vi "一体站氨氮总磷流程质控自动启动.vi"(6 "CODMn量程切换":enum32{"H", "L", "AUTO"}(ring)=enum."AUTO", 8 "总磷量程切换":enum32{"H", "L", "AUTO"}(ring)=enum."AUTO", 9 "总氮量程切换":enum32{"H", "L", "AUTO"}(ring)=enum."AUTO", 10 "氨氮量程切换":enum32{"H", "L", "AUTO"}(ring)=enum."AUTO", 11 "参数":T1={"是否启用仪器"=FALSE, "CODMn"={"启动测量模式"={"测量模式"=enum."水样测量"}, "确定按钮"=TRUE}, "启动模块"={"氨氮"=FALSE, "总磷"=FALSE, "总氮"=FALSE, "CODMn"=FALSE, "CODCr"=FALSE}, "常规启动"=FALSE, "直接启动"=FALSE}) -> ()   [LabVIEW 2016]
panel:
  out "枚举":enum16{"初始化", "采配水启动", "等待", "配水", "排水", "结束"}(ring)
  out "枚举 2":enum16{"初始化", "采配水启动", "等待", "配水", "排水", "结束"}(ring)
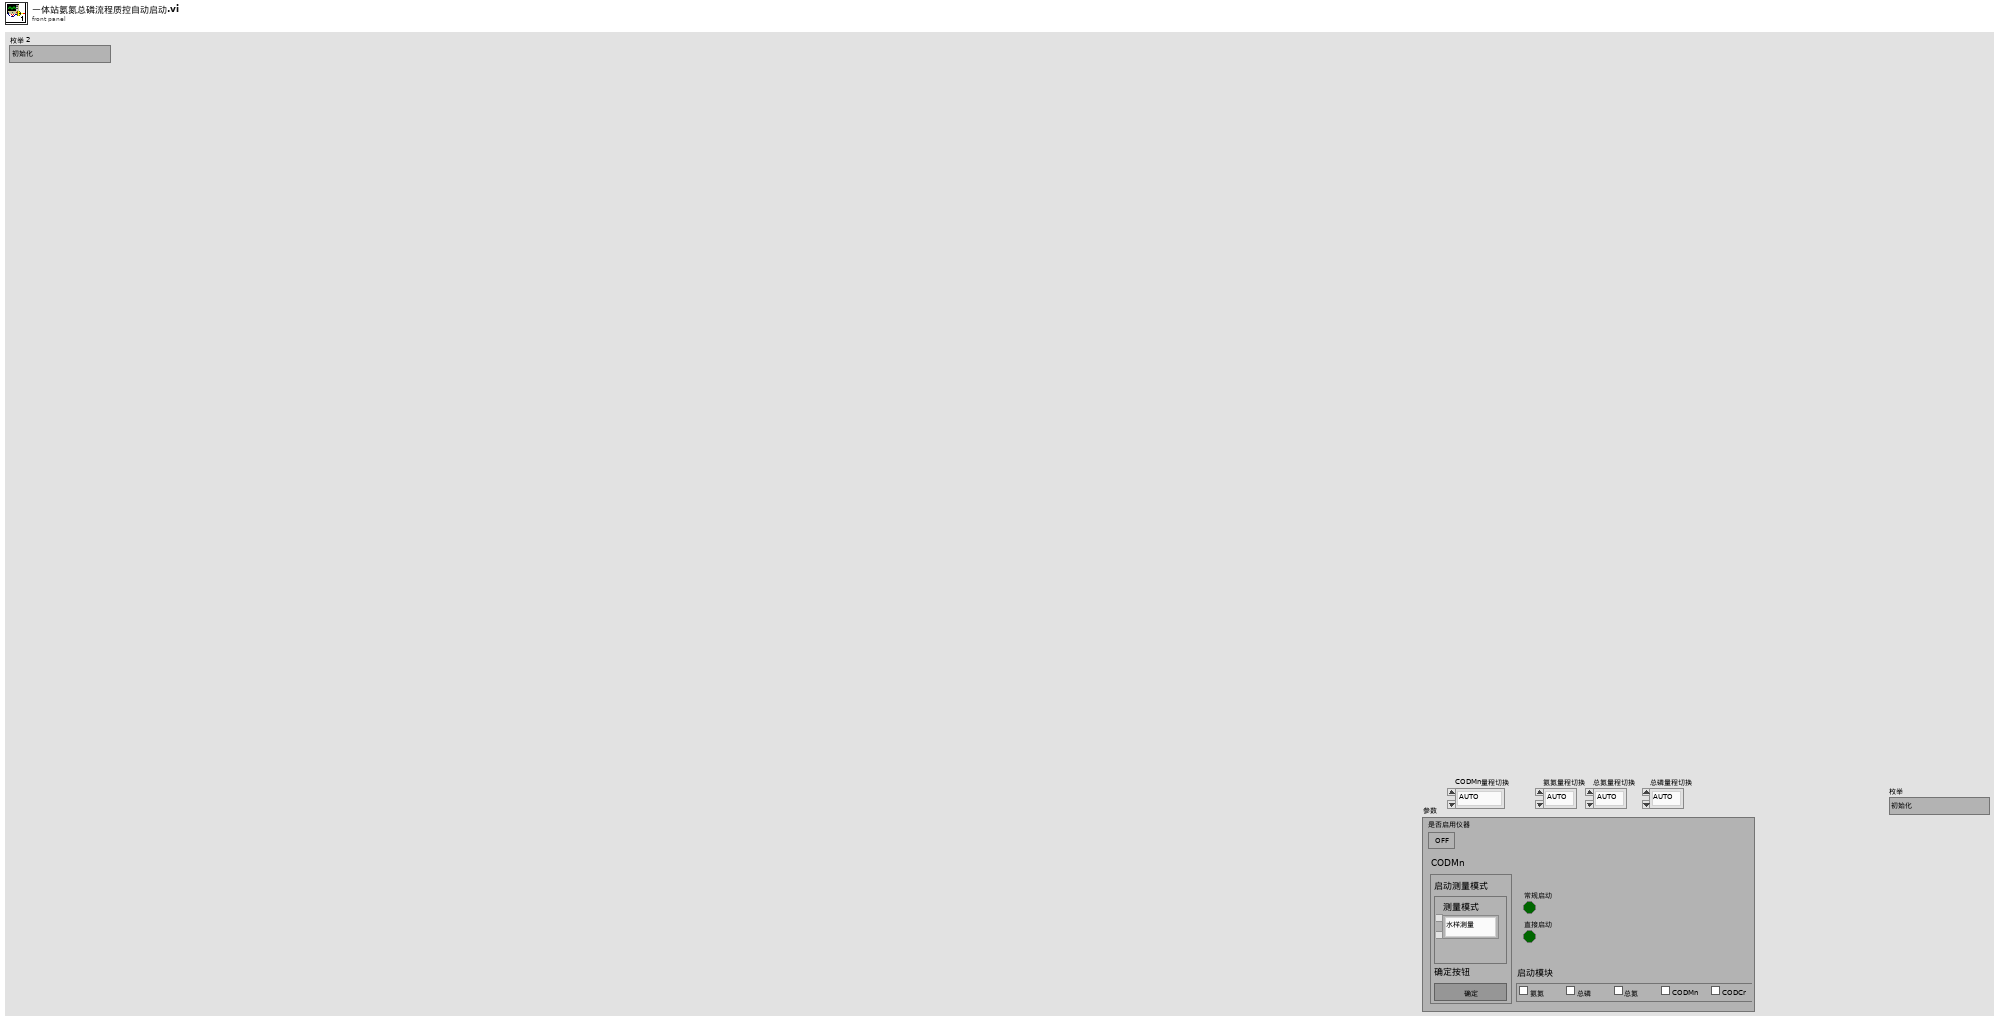
[diagram p1: front panel]
types:
  T1 = cluster{"是否启用仪器":bool, "CODMn":cluster{"启动测量模式":cluster{"测量模式":enum16{"水样测量", "标样核查", "加标回收", "平行样", "校零", "校标"}}, "确定按钮":bool}, "启动模块":cluster{"氨氮":bool, "总磷":bool, "总氮":bool, "CODMn":bool, "CODCr":bool}, "常规启动":bool, "直接启动":bool}
  T2 = cluster{"命令":string, cluster{"starting address":u16, "holding register value":u16}}
  T3 = cluster{"R0":i16, "R1":i16, "R2":i16, "R3":i16, "R4":i16, "R5":i16, "R6":i16, "R7":i16, "R8":i16, "R9":i16, "R10":i16, "R11":i16, "R12":i16, "R13":i16, "R14":i16, "R15":i16, "R16":i16, "R17":i16, "R18":i16, "R19":i16, "R20":i16, "R21":i16, "R22":i16, "R23":i16, "R24":i16, "R25":i16, "R26":i16, "R27":i16, "R28":i16, "R29":i16, "R30":i16, "R31":i16, "R32":i16, "R33":i16, "R34":i16, "R35":i16, "R36":i16, "R37":i16, "R38":i16, "R39":i16, "R40":i16, "R41":i16, "R42":i16, "R43":i16, "R44":i16, "R45":i16, "R46":i16, "R47":i16, "R48":i16, "R49":i16, "R50":i16, "R51":i16, "R52":i16, "R53":i16, "R54":i16, "R55":i16, "R56":i16}
  T4 = enum32{"Bad", "Idle", "Run top level", "Running"}
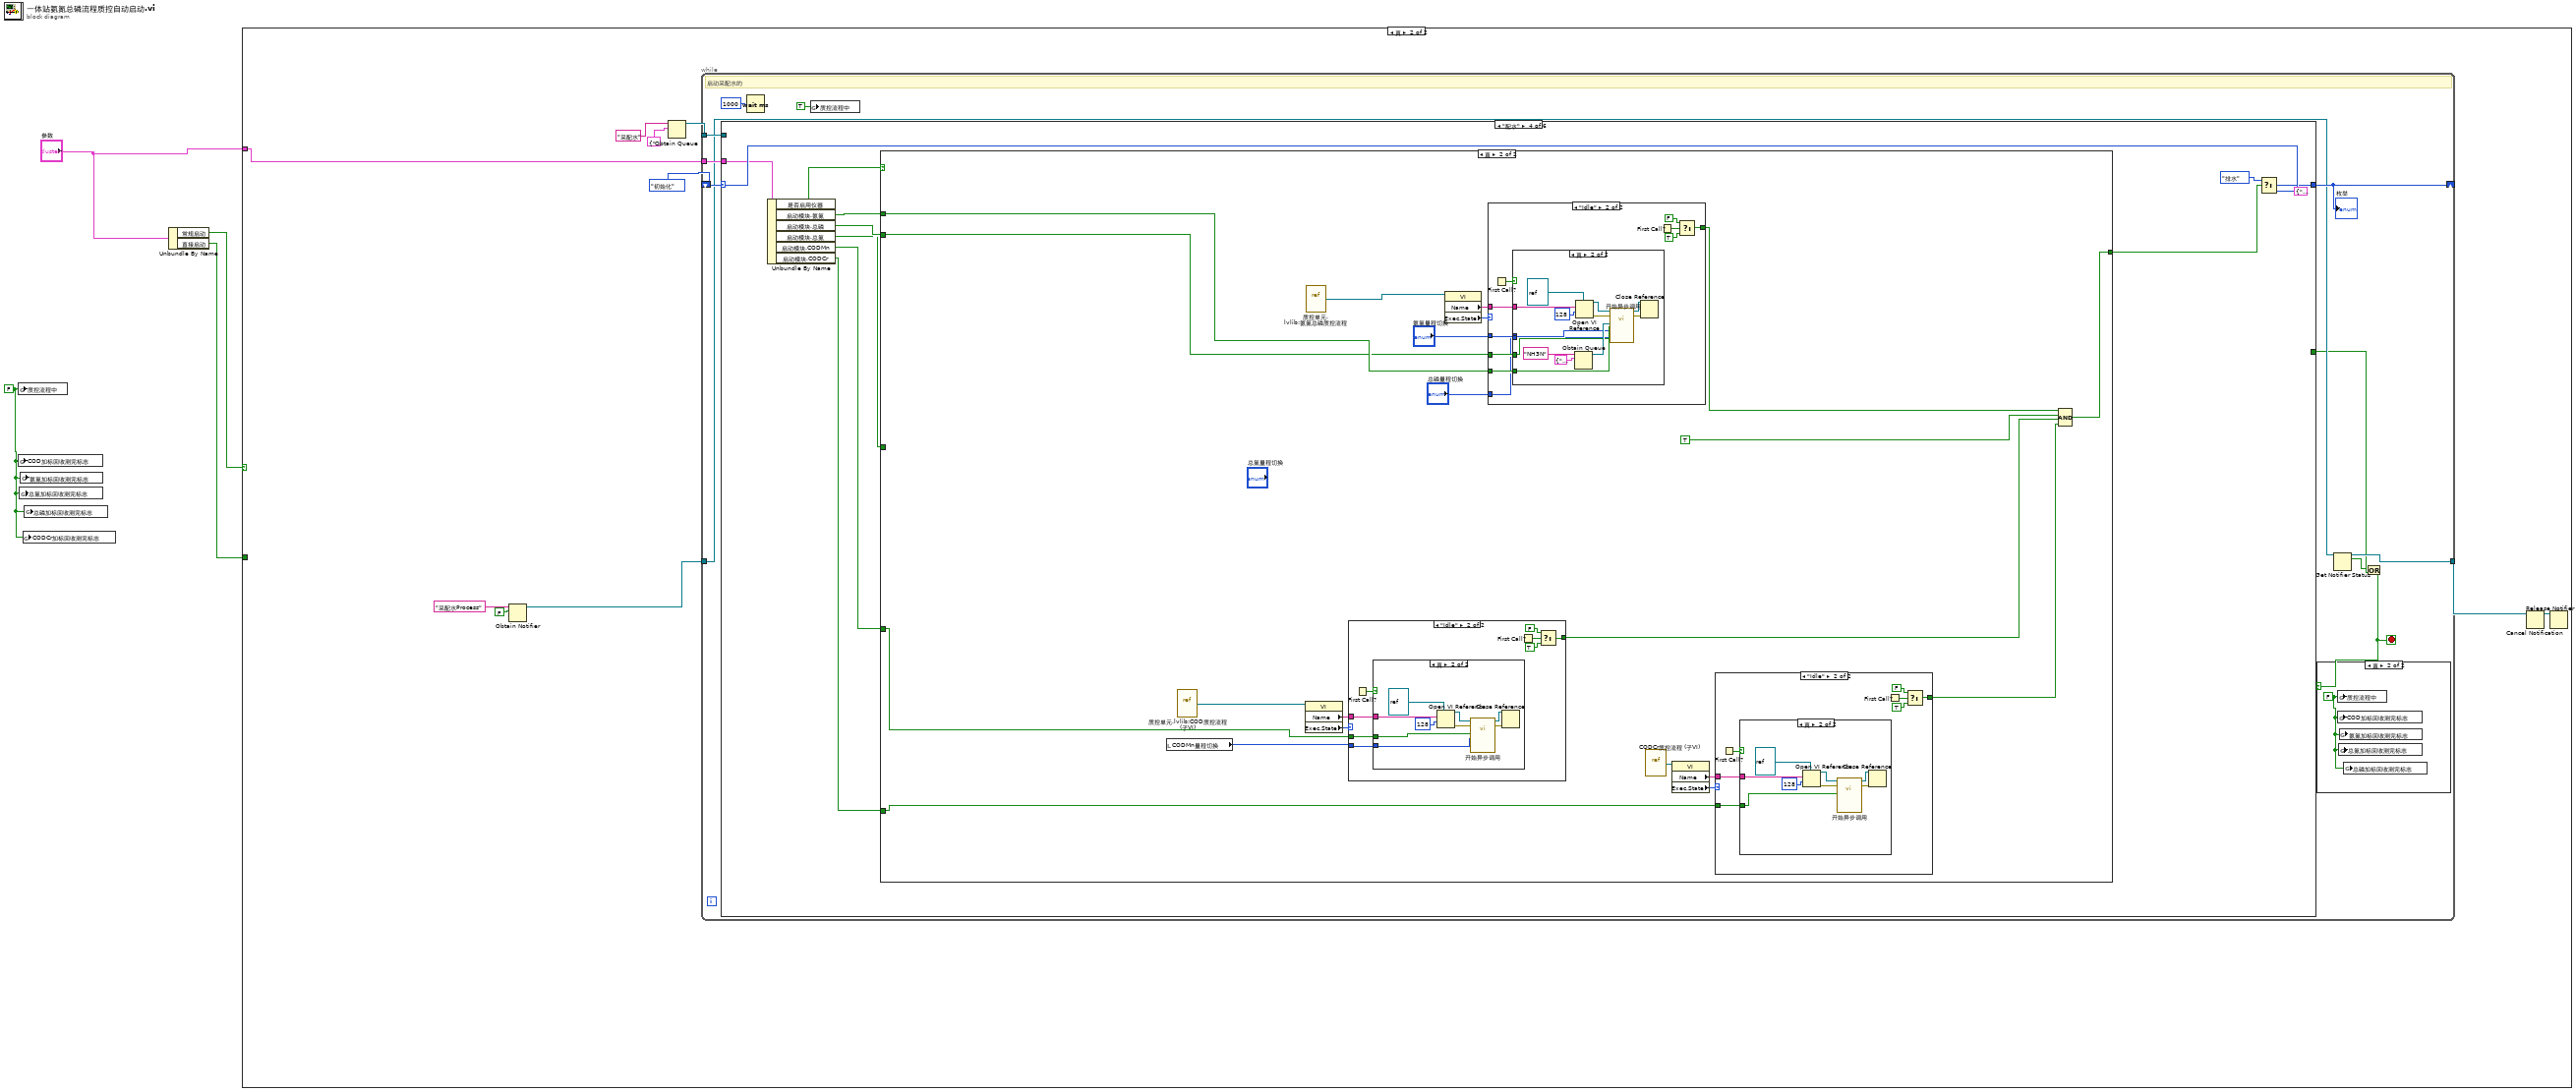
[diagram p0: block diagram]
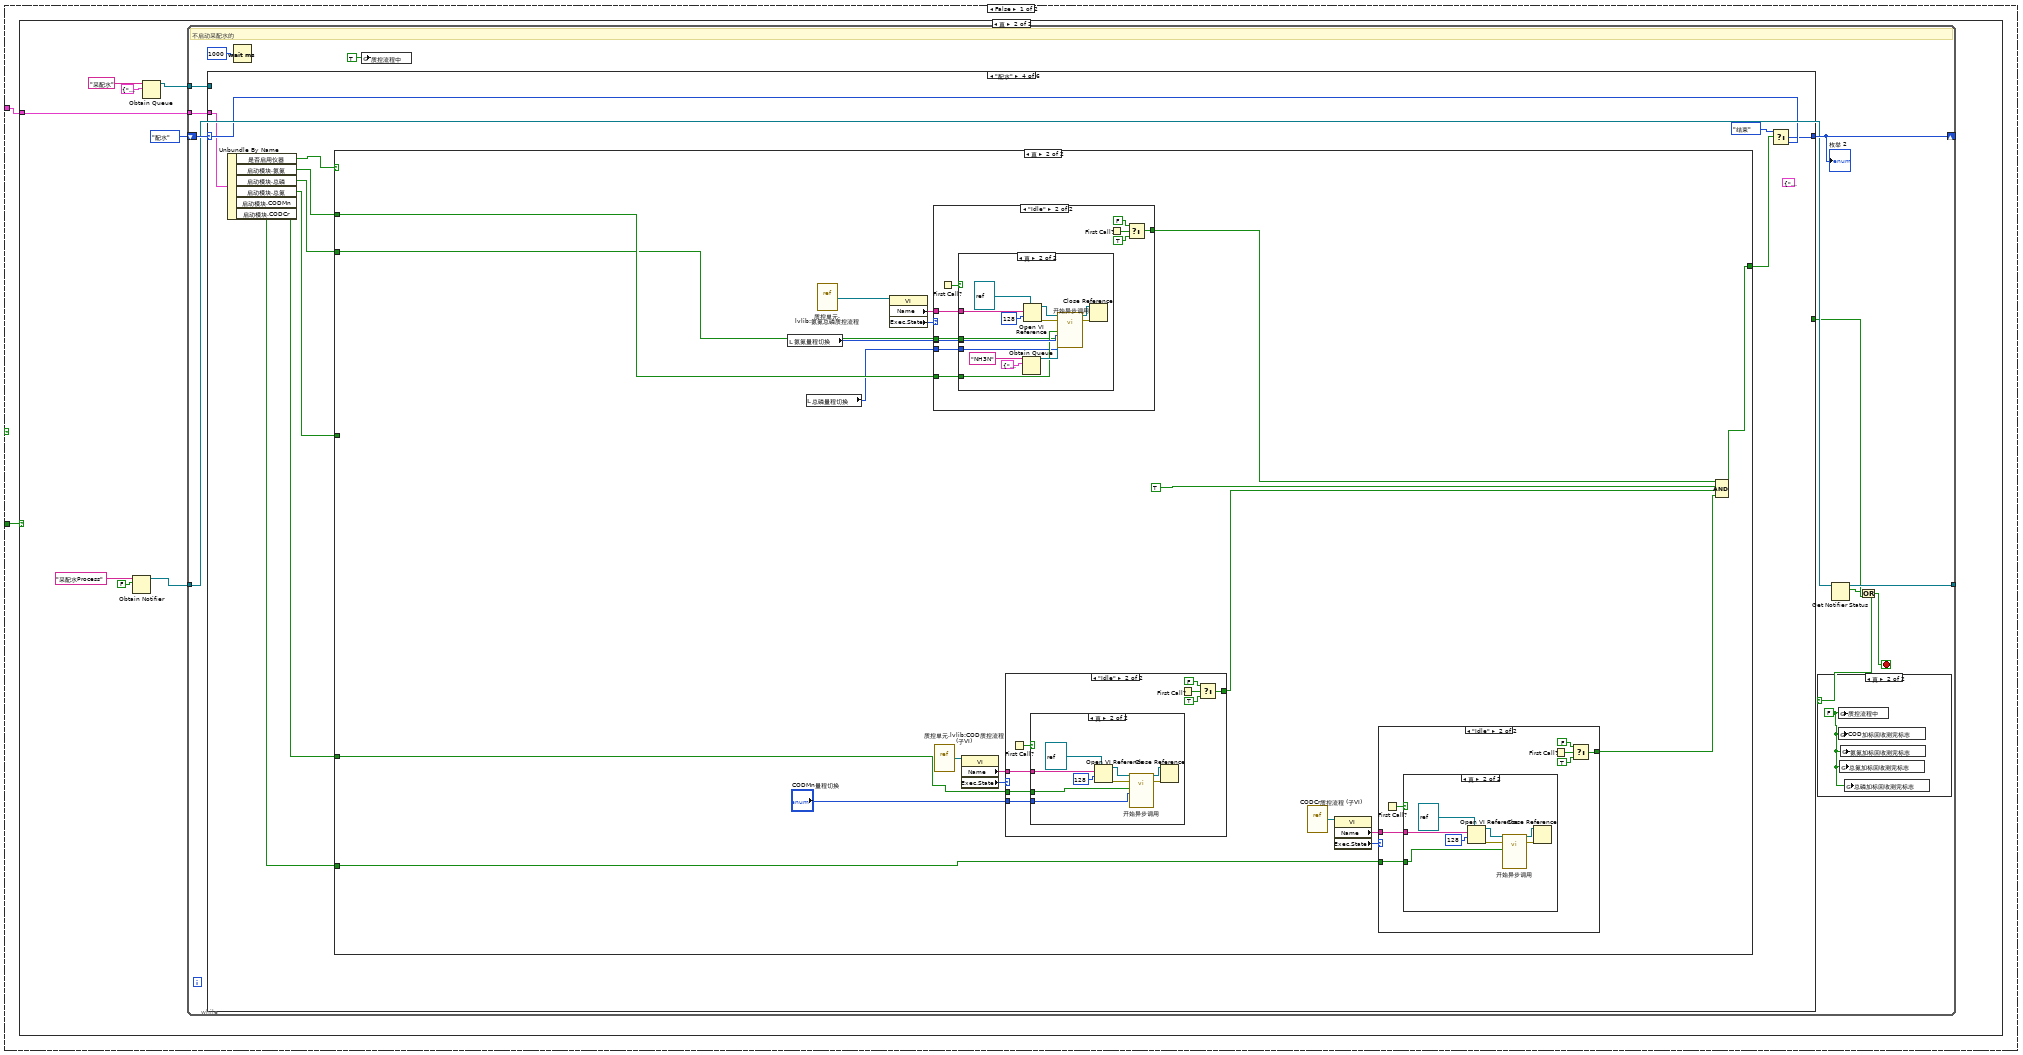
[diagram p2: hidden frame]
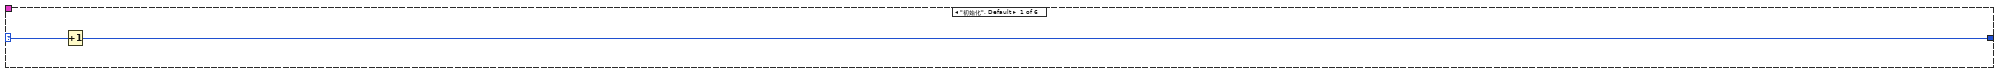
[diagram p5: hidden frame]
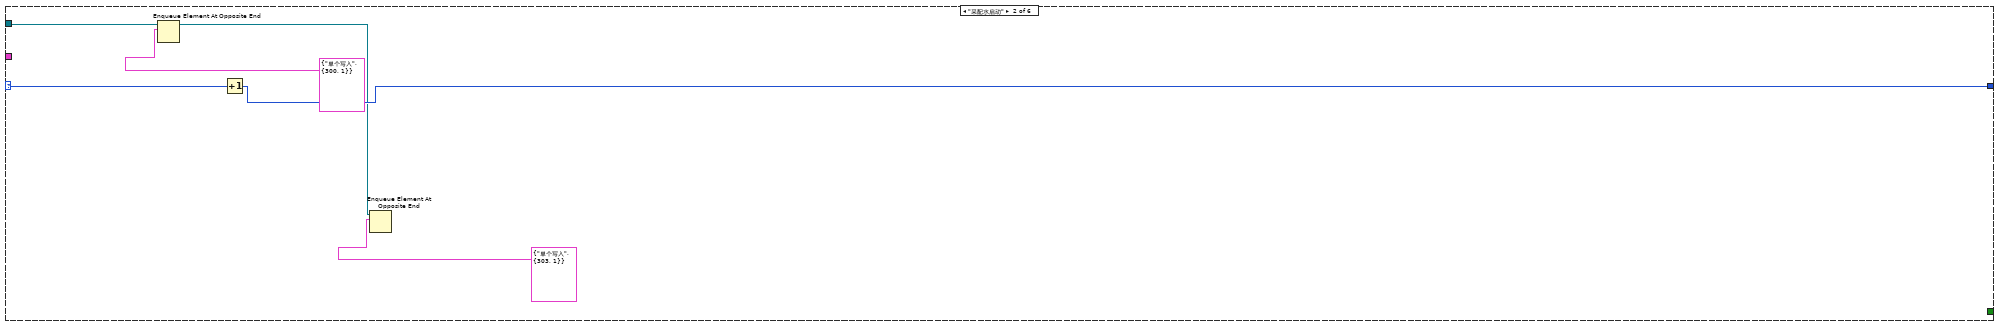
[diagram p6: hidden frame]
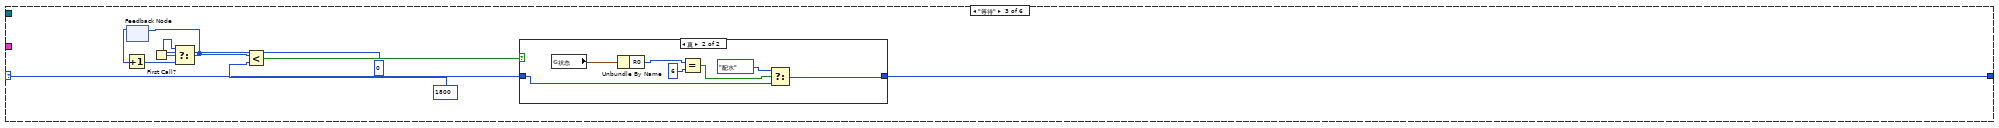
[diagram p7: hidden frame]
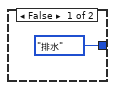
[diagram p8: hidden frame]
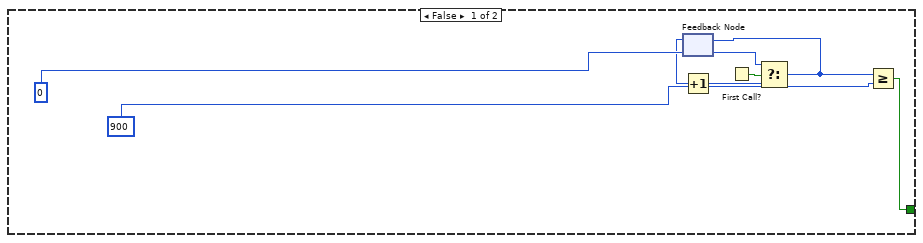
[diagram p9: hidden frame]
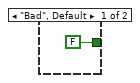
[diagram p10: hidden frame]
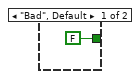
[diagram p12: hidden frame]
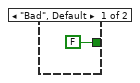
[diagram p14: hidden frame]
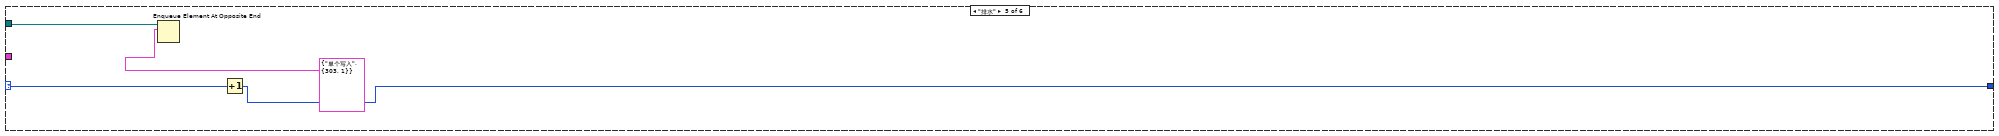
[diagram p16: hidden frame]
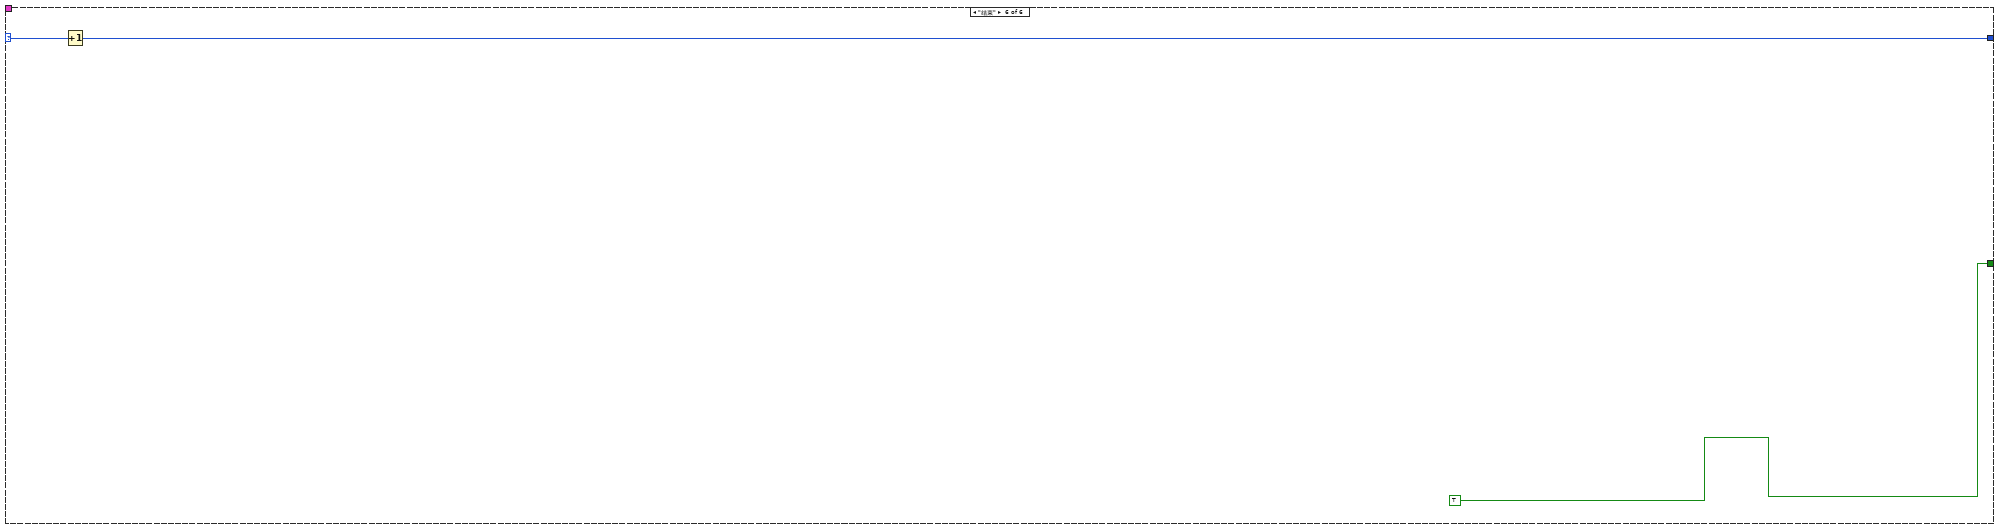
[diagram p17: hidden frame]
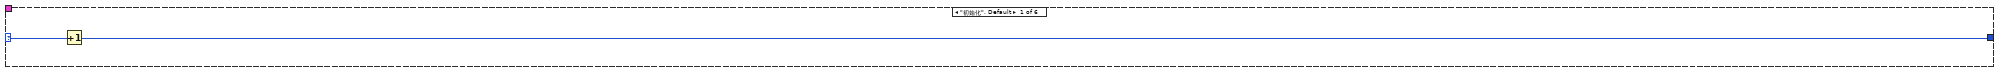
[diagram p19: hidden frame]
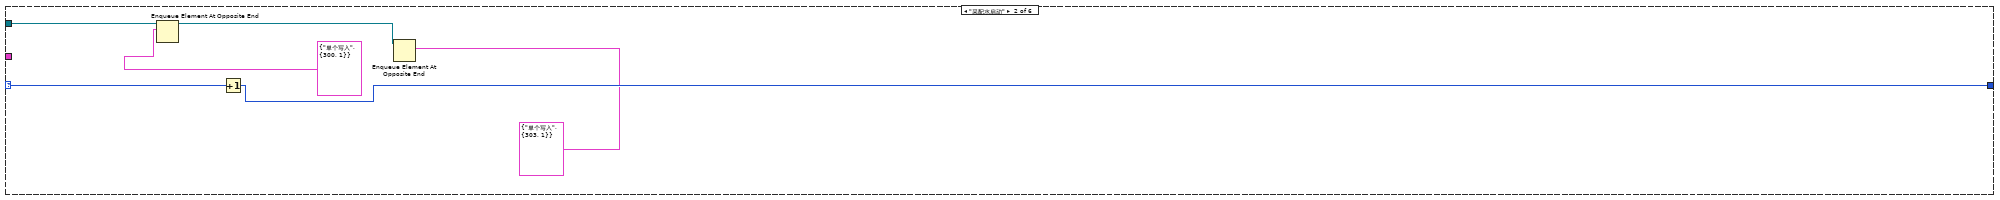
[diagram p20: hidden frame]
diagram:
  w1 = FALSE ("质控流程中")
  n1 = global write "质控测完标志全局 1.vi" "质控流程中"(w1) -> ()
  n2 = global write "质控测完标志全局 1.vi" "COD加标回收测完标志"(w1) -> ()
  n3 = global write "质控测完标志全局 1.vi" "总氮加标回收测完标志"(w1) -> ()
  n4 = global write "质控测完标志全局 1.vi" "氨氮加标回收测完标志"(w1) -> ()
  n5 = global write "质控测完标志全局 1.vi" "CODCr加标回收测完标志"(w1) -> ()
  n6 = global write "质控测完标志全局 1.vi" "总磷加标回收测完标志"(w1) -> ()
  n7 = Unbundle By Name("参数") -> ("常规启动"=w3:bool, "直接启动"=w2:bool)
  n8 = case shown="真" w3 {
    tunnel: "参数" -> [w5 w157]
    tunnel: w2 -> [w6 _]
    frame False {
      n9 = case shown="真" w6 {
        tunnel: w5 -> [_ w13]
        frame False {
        }
        frame True {
          n10 = Obtain Notifier(name (unnamed)="采配水Process" ("名称（未命名）"), notification data type=FALSE) -> (notifier out=w7:refnum<notifier>)  [unwired: 2 in, 2 out]
          n11 = Obtain Queue(name (unnamed)="采配水" ("名称（未命名）"), element data type=cluster{"命令":string, "数据":variant} {"命令"="", "数据"=variant}) -> (queue out=w10:refnum<queue>)  [unwired: 3 in, 2 out]
          n12 = while {
            tunnel: w10 -> [w25]
            shift-right: [w23] -> _
            shift-left: enum16{"初始化", "采配水启动", "等待", "配水", "排水", "结束"}."配水" ("枚举") -> [w24]
            tunnel: w13 -> [w21]
            tunnel: w7 -> [w20]
            tunnel: [w19] -> _
            stop <- w16 stop-if-true
            # "不启动采配水的"
            n13 = case shown="\"配水\"" w24 {
              selector: w24 -> [w28 w32 w41 w61 w151 w156]
              tunnel: w25 -> [_ w33 _ _ w152 _]
              tunnel: [w27 w31 w40 w60 w150 w155] -> w23
              tunnel: [_ _ _ _ _ TRUE] -> w18
              tunnel: w21 -> [_ _ _ w57 _ _]
              frame "初始化", Default {
                n14 = Increment(x=w28) -> (x+1=w27:enum16{"初始化", "采配水启动", "等待", "配水", "排水", "结束"})
              }
              frame "采配水启动" {
                n15 = Enqueue Element At Opposite End(queue=w33, element=T2 {"命令"="单个写入", {"starting address"=300, "holding register value"=1}} ("元素")) -> (queue out=w29:refnum<queue>)  [unwired: 2 in, 2 out]
                n16 = Increment(x=w32) -> (x+1=w31:enum16{"初始化", "采配水启动", "等待", "配水", "排水", "结束"})
                n17 = Enqueue Element At Opposite End(queue=w29, element=T2 {"命令"="单个写入", {"starting address"=303, "holding register value"=1}} ("元素")) -> ()  [unwired: 2 in, 3 out]
              }
              frame "等待" {
                n18 = feedback #1() -> (w37:i32)  [unwired: 1 in]
                n19 = Increment(x=w37) -> (x+1=w36:i32)
                n20 = First Call?() -> (First Call?: T/F=w38:bool)
                n21 = Select(t=0, s=w38, f=w36) -> (s? t:f=w35:i32)
                n22 = feedback-in #1(w35) -> ()
                n23 = Less?(x=w35, y=1800) -> (x < y?=w42:bool)
                n24 = case shown="真" w42 {
                  tunnel: w41 -> [_ w47]
                  tunnel: [enum16{"初始化", "采配水启动", "等待", "配水", "排水", "结束"}."排水" ("枚举") w46] -> w40
                  frame False {
                  }
                  frame True {
                    n25 = global read "与采配水交互全局.vi" "状态"() -> (w45:T3)
                    n26 = Unbundle By Name(w45) -> ("R0"=w51:i16)
                    n27 = Equal?(x=w51, y=i16 6) -> (x = y?=w49:bool)
                    n28 = Select(t=enum16{"初始化", "采配水启动", "等待", "配水", "排水", "结束"}."配水" ("枚举"), s=w49, f=w47) -> (s? t:f=w46:enum16{"初始化", "采配水启动", "等待", "配水", "排水", "结束"})
                  }
                }
              }
              frame "配水" {
                (unwired) cluster{"命令":string, "data":variant} {"命令"="启动", "data"=variant(cluster{"站号":u16, "控制命令输出":u16[]} {"站号"=1, "控制命令输出"=[256, 0]})} ("元素")
                n29 = Unbundle By Name(w57) -> ("是否启用仪器"=w59:bool, "启动模块.氨氮"=w55:bool, "启动模块.总磷"=w56:bool, "启动模块.总氮"=w53:bool, "启动模块.CODMn"=w54:bool, "启动模块.CODCr"=w52:bool)
                n30 = case shown="真" w59 {
                  tunnel: [w63 w90] -> w58
                  tunnel: w56 -> [_ w71]
                  tunnel: w55 -> [_ w86]
                  tunnel: w54 -> [_ w76]
                  tunnel: w53 -> [_ _]
                  tunnel: w52 -> [_ w73]
                  frame False {
                    n31 = feedback #2() -> (w67:i32)  [unwired: 1 in]
                    n32 = Increment(x=w67) -> (x+1=w66:i32)
                    n33 = First Call?() -> (First Call?: T/F=w68:bool)
                    n34 = Select(t=0, s=w68, f=w66) -> (s? t:f=w64:i32)
                    n35 = feedback-in #2(w64) -> ()
                    n36 = Greater Or Equal?(x=w64, y=900) -> (x >= y?=w63:bool)
                  }
                  frame True {
                    n37 = local read "氨氮量程切换"() -> (w84:enum32{"H", "L", "AUTO"})
                    n38 = local read "总磷量程切换"() -> (w70:enum32{"H", "L", "AUTO"})
                    n39 = vi-ref "质控单元.lvlib:氨氮总磷质控流程.vi"() -> (w88:refnum<vi>)
                    n40 = property class="VI"(reference=w88) -> ("Name"=w89:string, "Exec.State"=w87:T4)  [unwired: 1 in, 2 out]
                    n41 = case shown="\"Idle\"" w87 {
                      tunnel: w89 -> [_ w135]
                      tunnel: w86 -> [_ w134]
                      tunnel: [FALSE w129] -> w85
                      tunnel: w84 -> [_ w128]
                      tunnel: w71 -> [_ w127]
                      tunnel: w70 -> [_ w126]
                      frame "Bad", Default {
                      }
                      frame "Idle" {
                        n42 = First Call?() -> (First Call?: T/F=w133:bool)
                        n43 = case shown="真" w133 {
                          tunnel: w135 -> [_ w148]
                          tunnel: w134 -> [_ w138]
                          tunnel: w128 -> [_ w139]
                          tunnel: w127 -> [_ w137]
                          tunnel: w126 -> [_ w136]
                          frame False {
                          }
                          frame True {
                            n44 = Obtain Queue(name (unnamed)="NH3N" ("名称（未命名）"), element data type=cluster{"命令":string, "data":variant} {"命令"="", "data"=variant}) -> (queue out=w140:refnum<queue>)  [unwired: 3 in, 2 out]
                            n45 = Open VI Reference(type specifier VI Refnum (for type only)=refnum<vi> refnum ("类型说明符VI引用句柄（仅用于类型）"), vi path=w148, options=128 ("选项")) -> (vi reference=w149:refnum<vi>, error out=w145:errorcluster)  [unwired: 3 in]
                            n46 = call-by-ref "开始异步调用"(reference=w149, error in=w145, "队列输入"=w140, "氨氮"=w138, "氨氮量程切换"=w139, "总磷"=w137, "总磷量程切换"=w136) -> (reference out=w147:refnum<vi>, error out=w146:errorcluster)  [unwired: 8 in, 3 out]
                            n47 = Close Reference(reference=w147, error in (no error)=w146) -> ()  [unwired: 1 out]
                          }
                        }
                        n48 = First Call?() -> (First Call?: T/F=w132:bool)
                        n49 = Select(t=FALSE, s=w132, f=TRUE) -> (s? t:f=w129:bool)
                      }
                    }
                    n50 = vi-ref "质控单元.lvlib:COD质控流程 (子VI).vi"() -> (w81:refnum<vi>)
                    n51 = property class="VI"(reference=w81) -> ("Name"=w82:string, "Exec.State"=w80:T4)  [unwired: 1 in, 2 out]
                    n52 = case shown="\"Idle\"" w80 {
                      tunnel: w82 -> [_ w115]
                      tunnel: [FALSE w110] -> w74
                      tunnel: "CODMn量程切换" -> [_ w109]
                      tunnel: w76 -> [_ w108]
                      frame "Bad", Default {
                      }
                      frame "Idle" {
                        n53 = First Call?() -> (First Call?: T/F=w114:bool)
                        n54 = case shown="真" w114 {
                          tunnel: w115 -> [_ w123]
                          tunnel: w109 -> [_ w116]
                          tunnel: w108 -> [_ w117]
                          frame False {
                          }
                          frame True {
                            n55 = Open VI Reference(type specifier VI Refnum (for type only)=refnum<vi> refnum ("类型说明符VI引用句柄（仅用于类型）"), vi path=w123, options=128 ("选项")) -> (vi reference=w124:refnum<vi>, error out=w120:errorcluster)  [unwired: 3 in]
                            n56 = call-by-ref "开始异步调用"(reference=w124, error in=w120, "CODMn量程切换"=w116, "COD"=w117) -> (reference out=w122:refnum<vi>, error out=w121:errorcluster)  [unwired: 8 in, 2 out]
                            n57 = Close Reference(reference=w122, error in (no error)=w121) -> ()  [unwired: 1 out]
                          }
                        }
                        n58 = First Call?() -> (First Call?: T/F=w113:bool)
                        n59 = Select(t=FALSE, s=w113, f=TRUE) -> (s? t:f=w110:bool)
                      }
                    }
                    n60 = vi-ref "CODCr质控流程 (子VI).vi"() -> (w78:refnum<vi>)
                    n61 = property class="VI"(reference=w78) -> ("Name"=w79:string, "Exec.State"=w77:T4)  [unwired: 1 in, 2 out]
                    n62 = case shown="\"Idle\"" w77 {
                      tunnel: w79 -> [_ w98]
                      tunnel: [FALSE w93] -> w72
                      tunnel: w73 -> [_ w92]
                      frame "Bad", Default {
                      }
                      frame "Idle" {
                        n63 = First Call?() -> (First Call?: T/F=w97:bool)
                        n64 = case shown="真" w97 {
                          tunnel: w98 -> [_ w105]
                          tunnel: w92 -> [_ w99]
                          frame False {
                          }
                          frame True {
                            n65 = Open VI Reference(type specifier VI Refnum (for type only)=refnum<vi> refnum ("类型说明符VI引用句柄（仅用于类型）"), vi path=w105, options=128 ("选项")) -> (vi reference=w106:refnum<vi>, error out=w102:errorcluster)  [unwired: 3 in]
                            n66 = call-by-ref "开始异步调用"(reference=w106, error in=w102, "CODCr"=w99) -> (reference out=w104:refnum<vi>, error out=w103:errorcluster)  [unwired: 9 in, 2 out]
                            n67 = Close Reference(reference=w104, error in (no error)=w103) -> ()  [unwired: 1 out]
                          }
                        }
                        n68 = First Call?() -> (First Call?: T/F=w96:bool)
                        n69 = Select(t=FALSE, s=w96, f=TRUE) -> (s? t:f=w93:bool)
                      }
                    }
                    n70 = Compound Arithmetic op=AND ("复合运算")(w85, TRUE, w74, w72) -> (w90:bool)
                  }
                }
                n71 = Select(t=enum16{"初始化", "采配水启动", "等待", "配水", "排水", "结束"}."结束" ("枚举"), s=w58, f=w61) -> (s? t:f=w60:enum16{"初始化", "采配水启动", "等待", "配水", "排水", "结束"})
              }
              frame "排水" {
                n72 = Enqueue Element At Opposite End(queue=w152, element=T2 {"命令"="单个写入", {"starting address"=303, "holding register value"=1}} ("元素")) -> ()  [unwired: 2 in, 3 out]
                n73 = Increment(x=w151) -> (x+1=w150:enum16{"初始化", "采配水启动", "等待", "配水", "排水", "结束"})
              }
              frame "结束" {
                n74 = Increment(x=w156) -> (x+1=w155:enum16{"初始化", "采配水启动", "等待", "配水", "排水", "结束"})
              }
            }
            "枚举 2" <- w23
            n75 = Wait (ms)(milliseconds to wait=u32 1000 ("等待时间（毫秒）")) -> ()  [unwired: 1 out]
            n76 = global write "质控测完标志全局 1.vi" "质控流程中"(TRUE ("质控流程中")) -> ()
            n77 = Get Notifier Status(notifier=w20) -> (notifier out=w19:refnum<notifier>, current notification=w17:bool)  [unwired: 1 in, 3 out]
            n78 = Or(x=w17, y=w18) -> (x .or. y?=w16:bool)
            n79 = case shown="真" w16 {
              frame False {
              }
              frame True {
                w26 = FALSE ("质控流程中")
                n80 = global write "质控测完标志全局 1.vi" "质控流程中"(w26) -> ()
                n81 = global write "质控测完标志全局 1.vi" "COD加标回收测完标志"(w26) -> ()
                n82 = global write "质控测完标志全局 1.vi" "总氮加标回收测完标志"(w26) -> ()
                n83 = global write "质控测完标志全局 1.vi" "氨氮加标回收测完标志"(w26) -> ()
                n84 = global write "质控测完标志全局 1.vi" "总磷加标回收测完标志"(w26) -> ()
              }
            }
          }
        }
      }
    }
    frame True {
      n85 = Obtain Notifier(name (unnamed)="采配水Process" ("名称（未命名）"), notification data type=FALSE) -> (notifier out=w160:refnum<notifier>)  [unwired: 2 in, 2 out]
      n86 = Obtain Queue(name (unnamed)="采配水" ("名称（未命名）"), element data type=cluster{"命令":string, "数据":variant} {"命令"="", "数据"=variant}) -> (queue out=w164:refnum<queue>)  [unwired: 3 in, 2 out]
      n87 = while {
        tunnel: w164 -> [w177]
        shift-right: [w175] -> _
        shift-left: enum16{"初始化", "采配水启动", "等待", "配水", "排水", "结束"}."初始化" ("枚举") -> [w176]
        tunnel: w157 -> [w173]
        tunnel: w160 -> [w172]
        tunnel: [w171] -> w159
        stop <- w168 stop-if-true
        # "启动采配水的"
        n88 = case shown="\"配水\"" w176 {
          selector: w176 -> [w180 w184 w193 w213 w303 w308]
          tunnel: w177 -> [_ w185 _ _ w304 _]
          tunnel: [w179 w183 w192 w212 w302 w307] -> w175
          tunnel: [_ _ _ _ _ TRUE] -> w170
          tunnel: w173 -> [_ _ _ w209 _ _]
          frame "初始化", Default {
            n89 = Increment(x=w180) -> (x+1=w179:enum16{"初始化", "采配水启动", "等待", "配水", "排水", "结束"})
          }
          frame "采配水启动" {
            n90 = Enqueue Element At Opposite End(queue=w185, element=T2 {"命令"="单个写入", {"starting address"=300, "holding register value"=1}} ("元素")) -> (queue out=w182:refnum<queue>)  [unwired: 2 in, 2 out]
            n91 = Increment(x=w184) -> (x+1=w183:enum16{"初始化", "采配水启动", "等待", "配水", "排水", "结束"})
            n92 = Enqueue Element At Opposite End(queue=w182, element=T2 {"命令"="单个写入", {"starting address"=303, "holding register value"=1}} ("元素")) -> ()  [unwired: 2 in, 3 out]
          }
          frame "等待" {
            n93 = feedback #3() -> (w189:i32)  [unwired: 1 in]
            n94 = Increment(x=w189) -> (x+1=w188:i32)
            n95 = First Call?() -> (First Call?: T/F=w190:bool)
            n96 = Select(t=0, s=w190, f=w188) -> (s? t:f=w187:i32)
            n97 = feedback-in #3(w187) -> ()
            n98 = Less?(x=w187, y=1800) -> (x < y?=w194:bool)
            n99 = case shown="真" w194 {
              tunnel: w193 -> [_ w199]
              tunnel: [enum16{"初始化", "采配水启动", "等待", "配水", "排水", "结束"}."排水" ("枚举") w198] -> w192
              frame False {
              }
              frame True {
                n100 = global read "与采配水交互全局.vi" "状态"() -> (w197:T3)
                n101 = Unbundle By Name(w197) -> ("R0"=w203:i16)
                n102 = Equal?(x=w203, y=i16 6) -> (x = y?=w201:bool)
                n103 = Select(t=enum16{"初始化", "采配水启动", "等待", "配水", "排水", "结束"}."配水" ("枚举"), s=w201, f=w199) -> (s? t:f=w198:enum16{"初始化", "采配水启动", "等待", "配水", "排水", "结束"})
              }
            }
          }
          frame "配水" {
            (unwired) cluster{"命令":string, "data":variant} {"命令"="启动", "data"=variant(cluster{"站号":u16, "控制命令输出":u16[]} {"站号"=1, "控制命令输出"=[256, 0]})} ("元素")
            n104 = Unbundle By Name(w209) -> ("是否启用仪器"=w211:bool, "启动模块.氨氮"=w207:bool, "启动模块.总磷"=w208:bool, "启动模块.总氮"=w205:bool, "启动模块.CODMn"=w206:bool, "启动模块.CODCr"=w204:bool)
            n105 = case shown="真" w211 {
              tunnel: [w215 w242] -> w210
              tunnel: w208 -> [_ w223]
              tunnel: w207 -> [_ w237]
              tunnel: w206 -> [_ w227]
              tunnel: w205 -> [_ _]
              tunnel: w204 -> [_ w226]
              frame False {
                n106 = feedback #4() -> (w219:i32)  [unwired: 1 in]
                n107 = Increment(x=w219) -> (x+1=w218:i32)
                n108 = First Call?() -> (First Call?: T/F=w220:bool)
                n109 = Select(t=0, s=w220, f=w218) -> (s? t:f=w216:i32)
                n110 = feedback-in #4(w216) -> ()
                n111 = Greater Or Equal?(x=w216, y=900) -> (x >= y?=w215:bool)
              }
              frame True {
                n112 = local read "CODMn量程切换"() -> (w228:enum32{"H", "L", "AUTO"})
                n113 = vi-ref "质控单元.lvlib:COD质控流程 (子VI).vi"() -> (w233:refnum<vi>)
                n114 = property class="VI"(reference=w233) -> ("Name"=w234:string, "Exec.State"=w232:T4)  [unwired: 1 in, 2 out]
                n115 = vi-ref "质控单元.lvlib:氨氮总磷质控流程.vi"() -> (w240:refnum<vi>)
                n116 = case shown="\"Idle\"" w232 {
                  tunnel: w234 -> [_ w267]
                  tunnel: [FALSE w262] -> w225
                  tunnel: w228 -> [_ w261]
                  tunnel: w227 -> [_ w260]
                  frame "Bad", Default {
                  }
                  frame "Idle" {
                    n117 = First Call?() -> (First Call?: T/F=w266:bool)
                    n118 = case shown="真" w266 {
                      tunnel: w267 -> [_ w275]
                      tunnel: w261 -> [_ w268]
                      tunnel: w260 -> [_ w269]
                      frame False {
                      }
                      frame True {
                        n119 = Open VI Reference(type specifier VI Refnum (for type only)=refnum<vi> refnum ("类型说明符VI引用句柄（仅用于类型）"), vi path=w275, options=128 ("选项")) -> (vi reference=w276:refnum<vi>, error out=w272:errorcluster)  [unwired: 3 in]
                        n120 = call-by-ref "开始异步调用"(reference=w276, error in=w272, "CODMn量程切换"=w268, "COD"=w269) -> (reference out=w274:refnum<vi>, error out=w273:errorcluster)  [unwired: 8 in, 2 out]
                        n121 = Close Reference(reference=w274, error in (no error)=w273) -> ()  [unwired: 1 out]
                      }
                    }
                    n122 = First Call?() -> (First Call?: T/F=w265:bool)
                    n123 = Select(t=FALSE, s=w265, f=TRUE) -> (s? t:f=w262:bool)
                  }
                }
                n124 = property class="VI"(reference=w240) -> ("Name"=w241:string, "Exec.State"=w239:T4)  [unwired: 1 in, 2 out]
                n125 = case shown="\"Idle\"" w239 {
                  tunnel: w241 -> [_ w287]
                  tunnel: w237 -> [_ w286]
                  tunnel: [FALSE w281] -> w236
                  tunnel: "氨氮量程切换" -> [_ w280]
                  tunnel: w223 -> [_ w279]
                  tunnel: "总磷量程切换" -> [_ w278]
                  frame "Bad", Default {
                  }
                  frame "Idle" {
                    n126 = First Call?() -> (First Call?: T/F=w285:bool)
                    n127 = case shown="真" w285 {
                      tunnel: w287 -> [_ w300]
                      tunnel: w286 -> [_ w291]
                      tunnel: w280 -> [_ w290]
                      tunnel: w279 -> [_ w289]
                      tunnel: w278 -> [_ w288]
                      frame False {
                      }
                      frame True {
                        n128 = Obtain Queue(name (unnamed)="NH3N" ("名称（未命名）"), element data type=cluster{"命令":string, "data":variant} {"命令"="", "data"=variant}) -> (queue out=w292:refnum<queue>)  [unwired: 3 in, 2 out]
                        n129 = Open VI Reference(type specifier VI Refnum (for type only)=refnum<vi> refnum ("类型说明符VI引用句柄（仅用于类型）"), vi path=w300, options=128 ("选项")) -> (vi reference=w301:refnum<vi>, error out=w297:errorcluster)  [unwired: 3 in]
                        n130 = call-by-ref "开始异步调用"(reference=w301, error in=w297, "队列输入"=w292, "氨氮"=w291, "氨氮量程切换"=w290, "总磷"=w289, "总磷量程切换"=w288) -> (reference out=w299:refnum<vi>, error out=w298:errorcluster)  [unwired: 8 in, 3 out]
                        n131 = Close Reference(reference=w299, error in (no error)=w298) -> ()  [unwired: 1 out]
                      }
                    }
                    n132 = First Call?() -> (First Call?: T/F=w284:bool)
                    n133 = Select(t=FALSE, s=w284, f=TRUE) -> (s? t:f=w281:bool)
                  }
                }
                n134 = vi-ref "CODCr质控流程 (子VI).vi"() -> (w230:refnum<vi>)
                n135 = property class="VI"(reference=w230) -> ("Name"=w231:string, "Exec.State"=w229:T4)  [unwired: 1 in, 2 out]
                n136 = case shown="\"Idle\"" w229 {
                  tunnel: w231 -> [_ w250]
                  tunnel: [FALSE w245] -> w224
                  tunnel: w226 -> [_ w244]
                  frame "Bad", Default {
                  }
                  frame "Idle" {
                    n137 = First Call?() -> (First Call?: T/F=w249:bool)
                    n138 = case shown="真" w249 {
                      tunnel: w250 -> [_ w257]
                      tunnel: w244 -> [_ w251]
                      frame False {
                      }
                      frame True {
                        n139 = Open VI Reference(type specifier VI Refnum (for type only)=refnum<vi> refnum ("类型说明符VI引用句柄（仅用于类型）"), vi path=w257, options=128 ("选项")) -> (vi reference=w258:refnum<vi>, error out=w254:errorcluster)  [unwired: 3 in]
                        n140 = call-by-ref "开始异步调用"(reference=w258, error in=w254, "CODCr"=w251) -> (reference out=w256:refnum<vi>, error out=w255:errorcluster)  [unwired: 9 in, 2 out]
                        n141 = Close Reference(reference=w256, error in (no error)=w255) -> ()  [unwired: 1 out]
                      }
                    }
                    n142 = First Call?() -> (First Call?: T/F=w248:bool)
                    n143 = Select(t=FALSE, s=w248, f=TRUE) -> (s? t:f=w245:bool)
                  }
                }
                n144 = Compound Arithmetic op=AND ("复合运算")(w236, TRUE, w225, w224) -> (w242:bool)
              }
            }
            n145 = Select(t=enum16{"初始化", "采配水启动", "等待", "配水", "排水", "结束"}."排水" ("枚举"), s=w210, f=w213) -> (s? t:f=w212:enum16{"初始化", "采配水启动", "等待", "配水", "排水", "结束"})
          }
          frame "排水" {
            n146 = Enqueue Element At Opposite End(queue=w304, element=T2 {"命令"="单个写入", {"starting address"=303, "holding register value"=1}} ("元素")) -> ()  [unwired: 2 in, 3 out]
            n147 = Increment(x=w303) -> (x+1=w302:enum16{"初始化", "采配水启动", "等待", "配水", "排水", "结束"})
          }
          frame "结束" {
            n148 = Increment(x=w308) -> (x+1=w307:enum16{"初始化", "采配水启动", "等待", "配水", "排水", "结束"})
          }
        }
        "枚举" <- w175
        n149 = Wait (ms)(milliseconds to wait=u32 1000 ("等待时间（毫秒）")) -> ()  [unwired: 1 out]
        n150 = global write "质控测完标志全局 1.vi" "质控流程中"(TRUE ("质控流程中")) -> ()
        n151 = Get Notifier Status(notifier=w172) -> (notifier out=w171:refnum<notifier>, current notification=w169:bool)  [unwired: 1 in, 3 out]
        n152 = Or(x=w169, y=w170) -> (x .or. y?=w168:bool)
        n153 = case shown="真" w168 {
          frame False {
          }
          frame True {
            w178 = FALSE ("质控流程中")
            n154 = global write "质控测完标志全局 1.vi" "质控流程中"(w178) -> ()
            n155 = global write "质控测完标志全局 1.vi" "COD加标回收测完标志"(w178) -> ()
            n156 = global write "质控测完标志全局 1.vi" "总氮加标回收测完标志"(w178) -> ()
            n157 = global write "质控测完标志全局 1.vi" "氨氮加标回收测完标志"(w178) -> ()
            n158 = global write "质控测完标志全局 1.vi" "总磷加标回收测完标志"(w178) -> ()
          }
        }
      }
      n159 = Cancel Notification(0:w159) -> (8:w158:refnum<notifier>)  [unwired: 1 in, 2 out]
      n160 = Release Notifier(notifier=w158) -> ()  [unwired: 2 in, 3 out]
    }
  }
